vi "MES Tools.vi"(11 "Mes":T2) -> ()   [LabVIEW 2011]
uses:
  Button.ctl
panel:
  in  "停止":T1
  in  "选项卡控件":enum32{"用户校验测试", "上传测试结果", "手动上传结果"}(tab)
  in  "Login":T1
  in  "用户名":string
  in  "密码":string
  out "Upload Data-User":string="http://192.168.100.120:50000/manufacturing/IntegrationServlet?InterType=XML&message=<PRODUCTION_REQUEST><USER><SITE>A155</SITE><NAME>LTF</NAME><PWD>123456</PWD></USER></PRODUCTION_REQUEST>"
  out "RESULT":cluster{"Result":bool, "Message":string}
  in  "测试结果":string
  in  "合格？":bool
  out "Upload Data-Result":string="http://192.168.100.120:50000/manufacturing/IntegrationServlet?InterType=XML&message=<PRODUCTION_REQUEST><USER><SITE>A155</SITE><NAME>LTF</NAME><PWD>123456</PWD></USER></PRODUCTION_REQUEST>"
  in  "Login 2":T1
  in  "条码":string
  in  "Upload Data-Result Manu":string="http://192.168.100.120:50000/manufacturing/IntegrationServlet?InterType=XML&message=<PRODUCTION_REQUEST><USER><SITE>A155</SITE><NAME>LTF</NAME><PWD>123456</PWD></USER></PRODUCTION_REQUEST>"
  in  "Login 3":T1
  out "RESULT 3":cluster{"Result":bool, "Message":string} caption="RESULT"
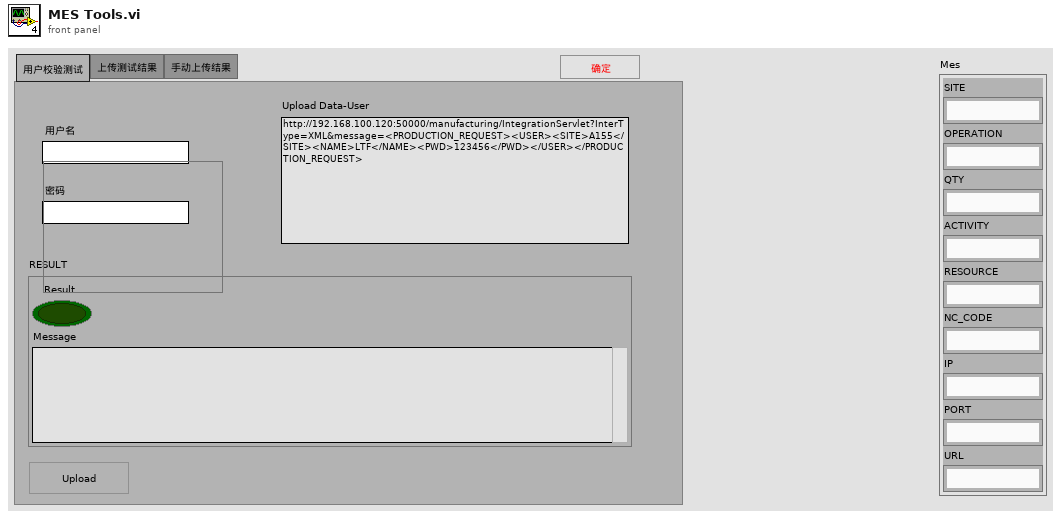
[diagram p1: front panel]
types:
  T1 = typedef "Button.ctl" = bool
  T2 = cluster{"SITE":string, "OPERATION":string, "QTY":string, "ACTIVITY":string, "RESOURCE":string, "NC_CODE":string, "IP":string, "PORT":string, "URL":string}
  T3 = typedef "MES设置.ctl" = cluster{"接口地址：":string, "SITE（站点）   ":string, "PWD（口令）":string, "RESOURCE（资源）":string, "OPERATION（工序）":string, "USER（用户）":string, "QTY":string, "ACTIVITY":string, "NC_CODE（NG代码）":string, "启用MES":bool}
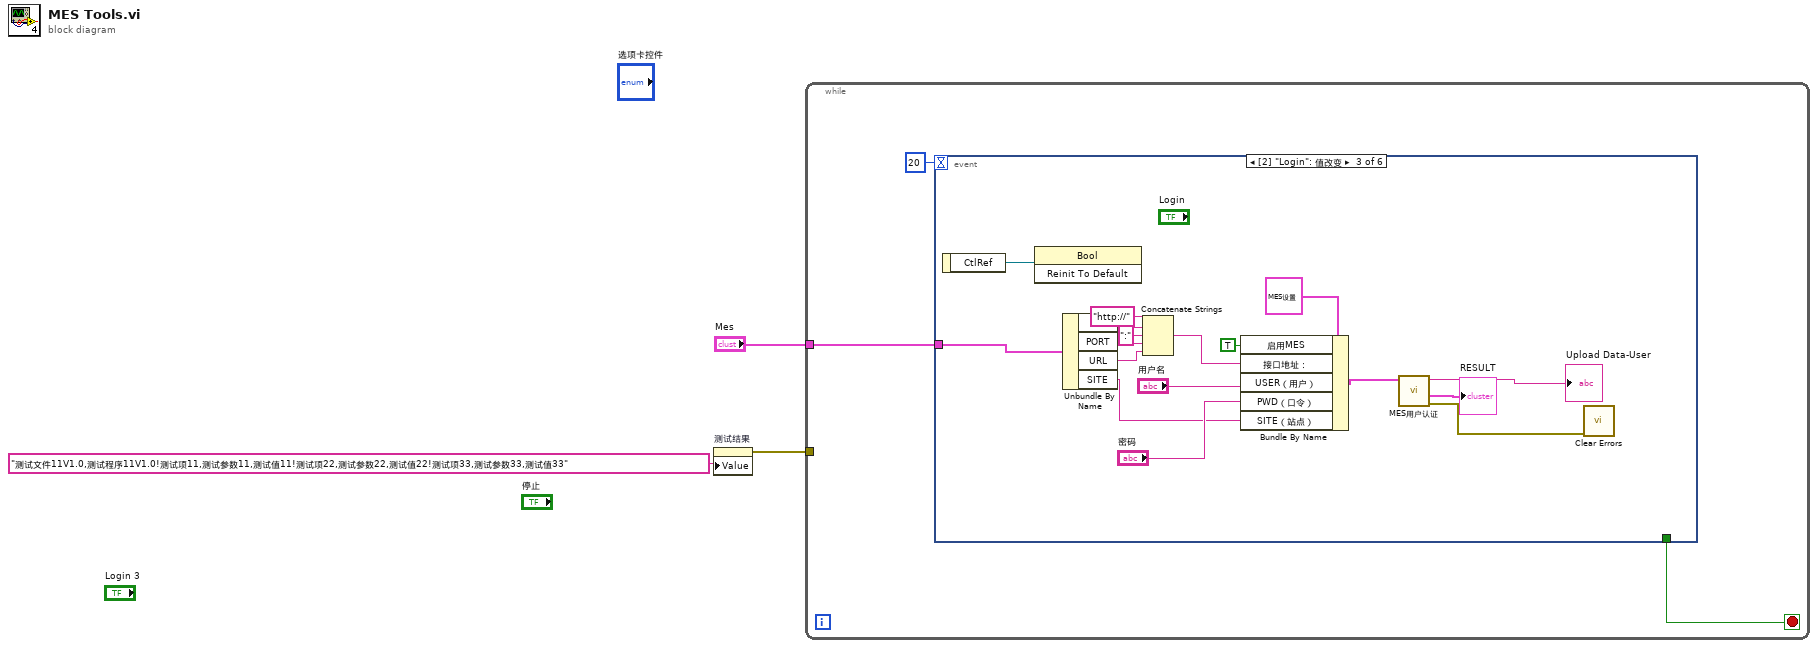
[diagram p0: block diagram]
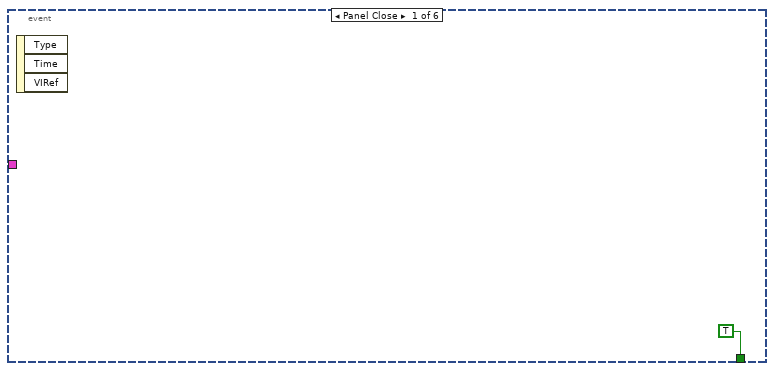
[diagram p2: hidden frame]
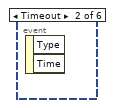
[diagram p3: hidden frame]
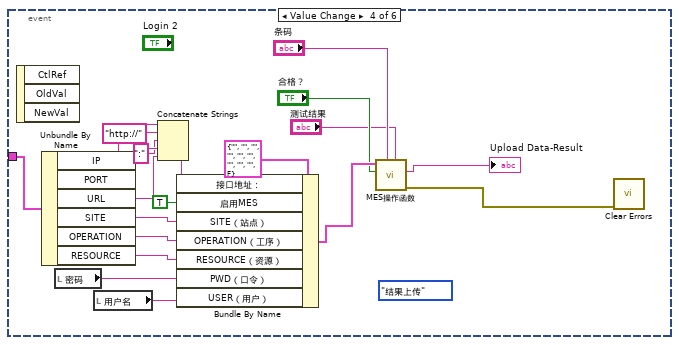
[diagram p4: hidden frame]
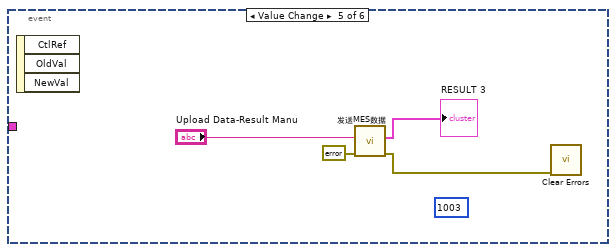
[diagram p5: hidden frame]
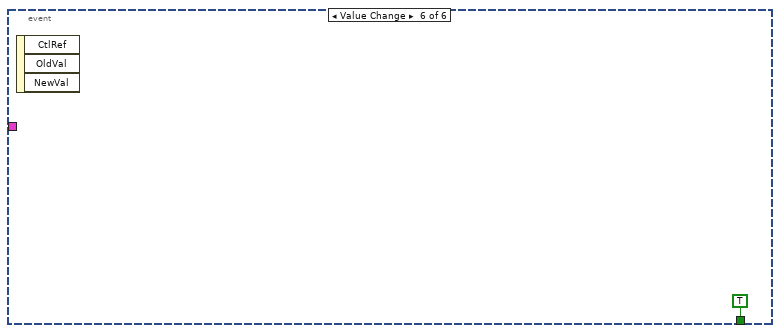
[diagram p6: hidden frame]
diagram:
  n1 = property on="测试结果" class="Str"("Value"="测试文件11V1.0,测试程序11V1.0!测试项11,测试参数11,测试值11!测试项22,测试参数22,测试值22!测试项33,测试参数33,测试值33") -> (error out=w2:errorcluster)  [unwired: 2 in, 1 out]
  n2 = while {
    tunnel: "Mes" -> [w4]
    tunnel: w2 -> [_]
    stop <- w5 stop-if-true
    n3 = event shown="[2] \"Login\": 值改变" {
      selector: _ -> [_ _ _ _ _ _]
      dyn-events: _ -> [_ _ _ _ _ _]
      timeout: 20 -> [_ _ _ _ _ _]
      tunnel: [TRUE _ _ _ _ TRUE] -> w5
      tunnel: w4 -> [_ _ w11 w33 _ _]
      event Panel Close {
        n4 = event-data() -> ()  [unwired: 1 in, 3 out]
      }
      event Timeout {
        n5 = event-data() -> ()  [unwired: 1 in, 2 out]
      }
      event Value Change {
        n6 = event-data() -> ("CtlRef"=w24:refnum<vi>)  [unwired: 1 in]
        n7 = invoke class="Bool" method="Reinit To Default"(reference=w24) -> ()  [unwired: 2 in, 3 out]
        n8 = Unbundle By Name(w11) -> ("IP"=w12:string, "PORT"=w15:string, "URL"=w16:string, "SITE"=w9:string)
        n9 = Concatenate Strings("http://" ("字符串"), w12, ":" ("字符串"), w15, w16) -> (w14:string)
        n10 = Bundle By Name(cluster=T3 {"接口地址："="http://192.168.18.1:50000/eeee", "SITE（站点）   "="", "PWD（口令）"="123456", "RESOURCE（资源）"="", "OPERATION（工序）"="", "USER（用户）"="Operator", "QTY"="", "ACTIVITY"="", "NC_CODE（NG代码）"="", "启用MES"=FALSE} ("MES配置"), "启用MES"=TRUE, "接口地址："=w14, "USER（用户）"="用户名", "PWD（口令）"="密码", "SITE（站点）"=w9) -> (w22:T3)
        n11 = call "MES用户认证.vi"("MES配置"=w22) -> ("error out"=w8:errorcluster, "RESULT"=→"RESULT":cluster{"Result":bool, "Message":string}, "Data(OUT)"=→"Upload Data-User":string)  [unwired: 8 in]
        n12 = call <vilib>:"Clear Errors.vi"("error in (no error)"=w8) -> ()  [unwired: 6 in, 1 out]
      }
      event Value Change {
        (unwired) enum16{"ID(SN)验证", "结果上传"}."结果上传" ("操作状态")
        n13 = event-data() -> ()  [unwired: 1 in, 3 out]
        n14 = Unbundle By Name(w33) -> ("IP"=w38:string, "PORT"=w36:string, "URL"=w37:string, "SITE"=w42:string, "OPERATION"=w40:string, "RESOURCE"=w41:string)
        n15 = local read "密码"() -> (w29:string)
        n16 = local read "用户名"() -> (w30:string)
        n17 = Concatenate Strings("http://" ("字符串"), w38, ":" ("字符串"), w36, w37) -> (w34:string)
        n18 = Bundle By Name(cluster=T3 {"接口地址："="", "SITE（站点）   "="", "PWD（口令）"="", "RESOURCE（资源）"="", "OPERATION（工序）"="", "USER（用户）"="", "QTY"="", "ACTIVITY"="", "NC_CODE（NG代码）"="", "启用MES"=FALSE} ("MES配置"), "接口地址："=w34, "启用MES"=TRUE, "SITE（站点）"=w42, "OPERATION（工序）"=w40, "RESOURCE（资源）"=w41, "PWD（口令）"=w29, "USER（用户）"=w30) -> (w31:T3)
        n19 = call "MES操作函数.vi"("测试结果"="测试结果", "SN"="条码", "总结果（测试）"="合格？", "MES配置"=w31) -> ("error out"=w25:errorcluster, "Data(OUT)"=→"Upload Data-Result":string)  [unwired: 5 in, 1 out]
        n20 = call <vilib>:"Clear Errors.vi"("error in (no error)"=w25) -> ()  [unwired: 6 in, 1 out]
      }
      event Value Change {
        (unwired) 1003 ("error code (no error:0)")
        n21 = event-data() -> ()  [unwired: 1 in, 3 out]
        n22 = call "发送MES数据.vi"("error in (no error)"=errorcluster {"status"=FALSE, "code"=0, "source"=""}, "Data(IN)"="Upload Data-Result Manu") -> ("error out"=w45:errorcluster, "RESULT"=→"RESULT 3":cluster{"Result":bool, "Message":string})  [unwired: 6 in, 2 out]
        n23 = call <vilib>:"Clear Errors.vi"("error in (no error)"=w45) -> ()  [unwired: 6 in, 1 out]
      }
      event Value Change {
        n24 = event-data() -> ()  [unwired: 1 in, 3 out]
      }
    }
  }
